vi "Create or Close PDF Document and PDFCopyr.vi"(0 "PDF Copy IN":refnum<k24>, 2 "Action":T3, 5 "PDF Document IN":refnum<k24>, 7 "File name":path, 11 "error in (no error)":errorcluster, 12 "PDF Details":T2, 13 "Permissions":T1={"User Password"="", "Owner Password"="", "Printing"=enum."Allow Printing", "Allow Modify Contents"=FALSE, "Allow Copy"=FALSE, "Allow Modify Annotations"=TRUE, "Allow Fill In "=TRUE, "Allow Screen Readers"=FALSE, "Allow Assembly"=FALSE}) -> (4 "PDF Copy OUT":refnum<k24>, 6 "PDF Document OUT":refnum<k24>, 15 "error out":errorcluster)   [LabVIEW 2019]
doc: "Version 1.0\nDeveloped by Jean-Marc Simard\nCopyright © 2012, Exaprom Inc.\nAll rights reserved.\nLicense: BSD\n\nWith iTextSharp Library\n(http://itextsharp.sourceforge.net)"
uses:
  <userlib>/Exaprom PDF/Controls/General Controls/Create or close.ctl
  C:/Program Files/National Instruments/LabVIEW 2019/user.lib/Exaprom PDF/DLL/itextsharp.dll
  DLL/itextsharp.dll
  <userlib>/Exaprom PDF/Controls/Initialization Controls/PDF Details.ctl
  <userlib>/Exaprom PDF/Controls/Initialization Controls/File Permission Parameters.ctl
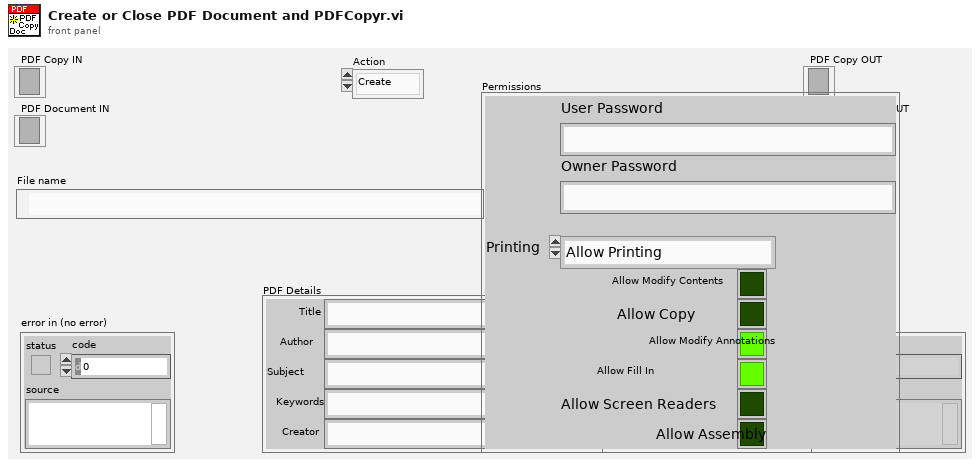
[diagram p1: front panel]
types:
  T1 = typedef "File Permission Parameters.ctl" = cluster{"User Password":string, "Owner Password":string, "Printing":enum16{"Allow Printing", "Allow Degraded Printing", "Don't Allow Printing"}, "Allow Modify Contents":bool, "Allow Copy":bool, "Allow Modify Annotations":bool, "Allow Fill In ":bool, "Allow Screen Readers":bool, "Allow Assembly":bool}
  T2 = typedef "PDF Details.ctl" = cluster{"Title":string, "Author":string, "Subject":string, "Keywords":string, "Creator":string}
  T3 = typedef "Create or close.ctl" = enum16{"Create", "Close"}
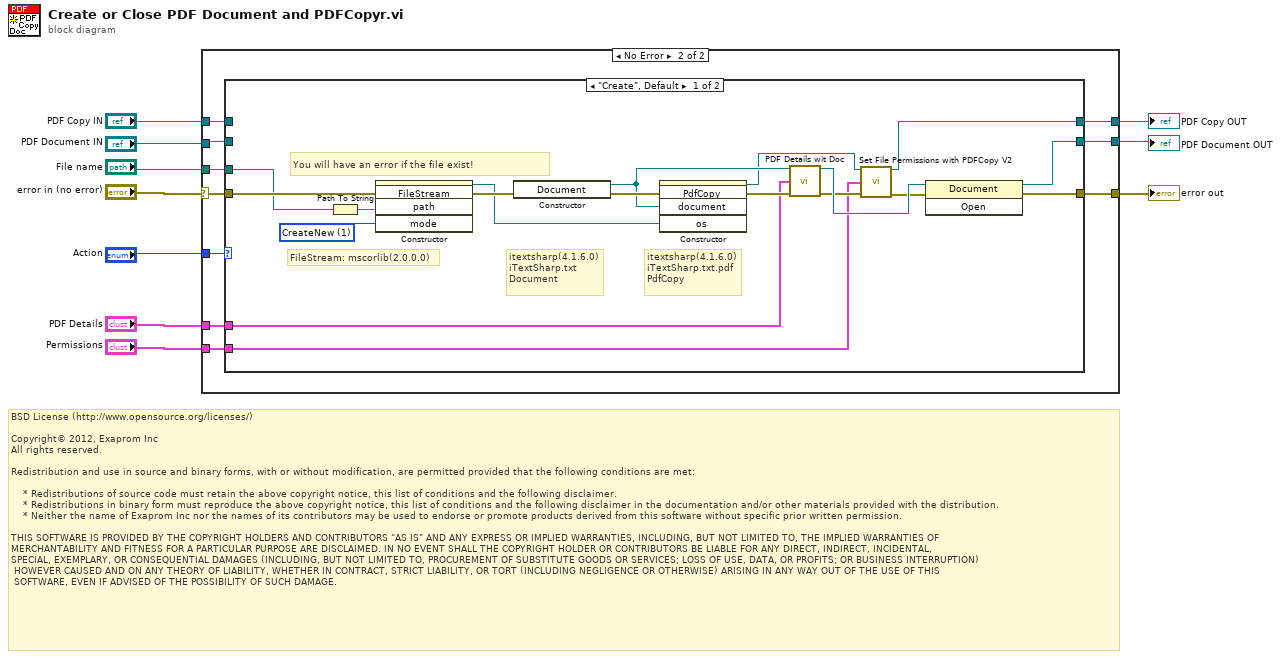
[diagram p0: block diagram]
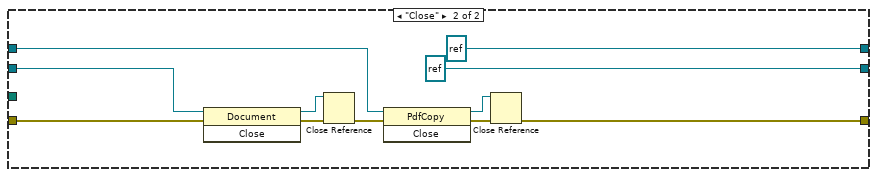
[diagram p3: hidden frame]
diagram:
  # "BSD License (http://www.opensource.org/licenses/)\n\nCopyright© 2012, Exaprom Inc\nAll rights reserved.\n\nRedistribution and use in source and binary forms, with or without modification, are permitted provided that the following conditions are met:\n\n    * Redistributions of source code must retain the above copyright notice, this list of conditions and the following disclaimer.\n    * Redistributions in binary form must reproduce the above copyright notice, this list of conditions and the following disclaimer in the documentation and/or other materials provided with the distribution.\n    * Neither the name of Exaprom Inc nor the names of its contributors may be used to endorse or promote products derived from this software without specific prior written permission.\n\nTHIS SOFTWARE IS PROVIDED BY THE COPYRIGHT HOLDERS AND CONTRIBUTORS \"AS IS\" AND ANY EXPRESS OR IMPLIED WARRANTIES, INCLUDING, BUT NOT LIMITED TO, THE IMPLIED WARRANTIES OF \nMERCHANTABILITY AND FITNESS FOR A PARTICULAR PURPOSE ARE DISCLAIMED. IN NO EVENT SHALL THE COPYRIGHT HOLDER OR CONTRIBUTORS BE LIABLE FOR ANY DIRECT, INDIRECT, INCIDENTAL,\nSPECIAL, EXEMPLARY, OR CONSEQUENTIAL DAMAGES (INCLUDING, BUT NOT LIMITED TO, PROCUREMENT OF SUBSTITUTE GOODS OR SERVICES; LOSS OF USE, DATA, OR PROFITS; OR BUSINESS INTERRUPTION)\n HOWEVER CAUSED AND ON ANY THEORY OF LIABILITY, WHETHER IN CONTRACT, STRICT LIABILITY, OR TORT (INCLUDING NEGLIGENCE OR OTHERWISE) ARISING IN ANY WAY OUT OF THE USE OF THIS\n SOFTWARE, EVEN IF ADVISED OF THE POSSIBILITY OF SUCH DAMAGE."
  n1 = case shown="No Error" "error in (no error)" {
    selector: "error in (no error)" -> [w13 w23]
    tunnel: [w13 w20] -> w10
    tunnel: "File name" -> [_ w22]
    tunnel: "Action" -> [_ w21]
    tunnel: [w12 w19] -> w4
    tunnel: [w11 w18] -> w3
    tunnel: "PDF Copy IN" -> [w12 w17]
    tunnel: "PDF Document IN" -> [w11 w16]
    tunnel: "PDF Details" -> [_ w15]
    tunnel: "Permissions" -> [_ w14]
    frame Error {
    }
    frame No Error {
      n2 = case shown="\"Create\", Default" w21 {
        tunnel: w23 -> [w39 w45]
        tunnel: w22 -> [w38 _]
        tunnel: [w26 refnum<k24> refnum ("new reference")] -> w19
        tunnel: [w34 refnum<k24> refnum ("new reference")] -> w18
        tunnel: [w33 w42] -> w20
        tunnel: w17 -> [_ w47]
        tunnel: w16 -> [_ w46]
        tunnel: w15 -> [w25 _]
        tunnel: w14 -> [w24 _]
        frame "Create", Default {
          w41 = 1 items=["CreateNew"=1, "Create"=2, "Open"=3, "OpenOrCreate"=4, "Truncate"=5, "Append"=6] ("mode")
          # "itextsharp(4.1.6.0)\niTextSharp.txt.pdf\nPdfCopy"
          # "itextsharp(4.1.6.0)\niTextSharp.txt\nDocument"
          # "You will have an error if the file exist!"
          # "FileStream: mscorlib(2.0.0.0)"
          n3 = Path To String(path=w38) -> (string=w40:string)
          n4 = constructor class="FileStream" ("Constructor Node")(error in=w39, "path"=w40, "mode"=w41) -> (reference out=w35:refnum<k24>, error out=w36:errorcluster)  [unwired: 2 in, 3 out]
          n5 = constructor class="Document"(error in=w36) -> (reference out=w31:refnum<k24>, error out=w37:errorcluster)  [unwired: 2 in, 1 out]
          n6 = constructor class="PdfCopy"(error in=w37, "document"=w31, "os"=w35) -> (reference out=w27:refnum<k24>, error out=w32:errorcluster)  [unwired: 2 in, 3 out]
          n7 = call <userlib>:"PDF Details wit Doc.vi"("PDF Document IN"=w31, "PDF Details"=w25, "error in (no error)"=w32) -> ("PDF Document OUT"=w30:refnum<k24>, "error out"=w29:errorcluster)  [unwired: 11 in]
          n8 = call <userlib>:"Set File Permissions with PDFCopy V2.vi"("PDF Copy IN"=w27, "Permissions"=w24, "error in (no error)"=w29) -> ("PDF Copy OUT"=w26:refnum<k24>, "error out"=w28:errorcluster)  [unwired: 11 in]
          n9 = invoke class="Document" method="Open"(reference=w30, error in=w28) -> (reference out=w34:refnum<k24>, error out=w33:errorcluster)  [unwired: 1 in, 1 out]
        }
        frame "Close" {
          n10 = invoke class="Document" method="Close"(reference=w46, error in=w45) -> (reference out=w49:refnum<k24>, error out=w48:errorcluster)  [unwired: 1 in, 1 out]
          n11 = Close Reference(reference=w49, error in (no error)=w48) -> (error out=w50:errorcluster)
          n12 = invoke class="PdfCopy" method="Close"(reference=w47, error in=w50) -> (reference out=w52:refnum<k24>, error out=w51:errorcluster)  [unwired: 1 in, 1 out]
          n13 = Close Reference(reference=w52, error in (no error)=w51) -> (error out=w42:errorcluster)
        }
      }
    }
  }
  "error out" <- w10
  "PDF Copy OUT" <- w4
  "PDF Document OUT" <- w3
